vi "RT - Process Time Out.vi"(4 "Action Stop":variant, 5 "Message Queue":refnum<queue>, 6 "Action In":variant, 7 "Timeout & Advice":T1, 8 "Error In":errorcluster, 9 "Counts":i32, 10 "Fs (Hz)":dbl=100.0, 11 "Duration (Sec)":dbl=20.0) -> (0 "Error Out":errorcluster, 3 "Action Out":variant)   [LabVIEW 2016]
uses:
  Message Queue/Message Cluster.ctl
  Message Queue/Message.ctl
  Controls/Timeout Message.ctl
  Controls/Status Message.ctl
  Message Queue/Message Queue.lvlib
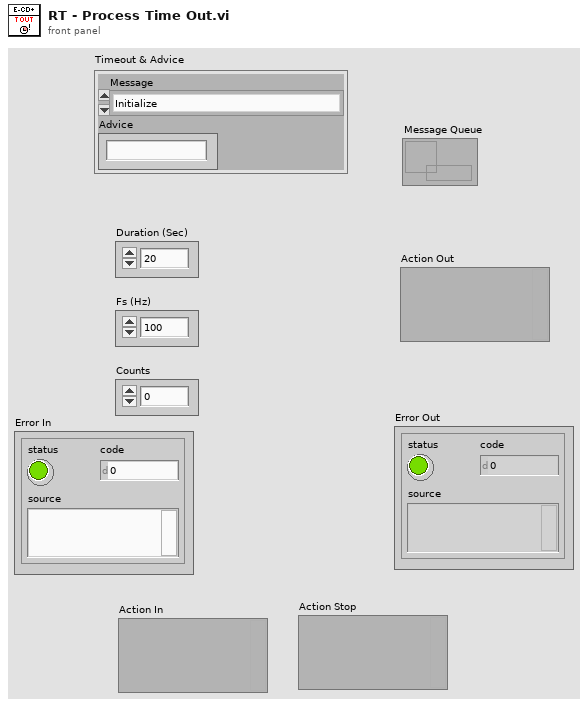
[diagram p1: front panel]
types:
  T1 = typedef "Timeout Message.ctl" = cluster{"Message":T2, "Advice":string}
  T2 = typedef "Message Queue.lvlib/Message.ctl" = enum16{"Initialize", "Initialize UI Refs", "Disable Controls", "Enable UI Controls", "Connect RT", "Get Control Mode from RT", "Send Control Mode to UI", "Update Control Mode", "Get Config from RT", "Send Config to UI", "Update Parameters", "Change Parameters", "Calibrate Config", "Update Calibration", "Change Valve State", "Get Valve Status from RT", "Send Valve Status to UI", "Update Valve Status", "Inital UI Values", "Disconnect RT", "Close Connection", "Disconnect UI", "Run Mode", "Stop ALL", "Change Control Mode", "Skid Manual", "Computer Manual", "Step Automated", "Fully Automated", "Reset", "Critical Error", "Log-Only Error", "Non-Critical Error", "RT Error", "Update System Status", "Update DI Status", "Clear System Status", "Update Warning", "Clear Warning", "Upate Timeout", "Update Reset Status", "Waiting", "Verify Password", "Manual Cleaning Process", "Update Manual Cleaning Process", "Exit", "---Copy This Frame---"}
  T3 = typedef "Status Message.ctl" = cluster{"Message":string, "Step #":i32, "Start/End":bool}
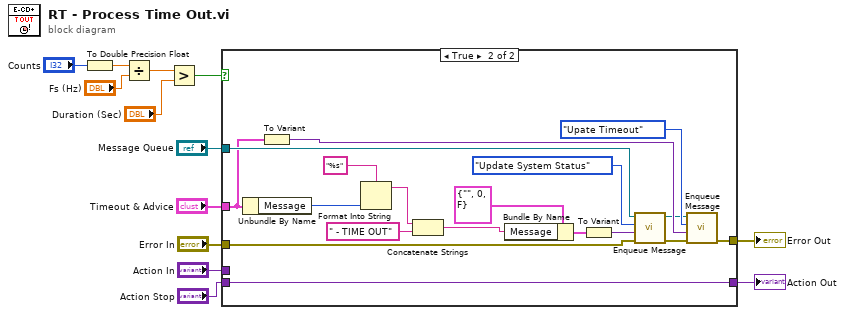
[diagram p0: block diagram]
diagram:
  n1 = To Double Precision Float(number="Counts") -> (double precision float=w9:dbl)
  n2 = Divide(x=w9, y="Fs (Hz)") -> (x/y=w11:dbl)
  n3 = Greater?(x=w11, y="Duration (Sec)") -> (0:w8:bool)
  n4 = case shown="True" w8 {
    tunnel: "Message Queue" -> [_ w29]
    tunnel: "Timeout & Advice" -> [_ w17]
    tunnel: "Action In" -> [w15 _]
    tunnel: "Action Stop" -> [_ w31]
    tunnel: [w15 w31] -> w4
    tunnel: "Error In" -> [w14 w27]
    tunnel: [w14 w30] -> w2
    frame False {
    }
    frame True {
      n5 = Unbundle By Name(w17) -> ("Message"=w16:T2)
      n6 = To Variant(anything=w17) -> (Variant=w32:variant)
      n7 = Format Into String(format string="%s", w16) -> (resulting string=w19:string)  [unwired: 2 in, 1 out]
      n8 = Concatenate Strings(w19, " - TIME OUT" ("string")) -> (w18:string)
      n9 = Bundle By Name(cluster=T3 {"Message"="", "Step #"=0, "Start/End"=FALSE} ("Status Message"), "Message"=w18) -> (w23:T3)
      n10 = To Variant(anything=w23) -> (Variant=w22:variant)
      n11 = call "Enqueue Message.vi"("error in (no error)"=w27, "Message Data"=w22, "Message"=Message."Update System Status", "Message Queue"=w29) -> ("error out"=w26:errorcluster, "dup Message Queue"=w28:refnum<queue>)  [unwired: 6 in]
      n12 = call "Enqueue Message.vi"("error in (no error)"=w26, "Message Data"=w32, "Message"=Message."Upate Timeout", "Message Queue"=w28) -> ("error out"=w30:errorcluster)  [unwired: 6 in, 1 out]
    }
  }
  "Action Out" <- w4
  "Error Out" <- w2
